vi "波形生成与数据存储.vi"(6 "文件保存控制位":bool, 9 "数据输入":i32[][](array[numeric]), 10 "上一时刻时间输入":timestamp, 11 "文件存储地址":path) -> (1 "缓存区输出":i32[][](array[numeric]), 2 "时间输出":timestamp, 3 "波形图表 6":waveform(i32)[](graph))   [LabVIEW 2020]
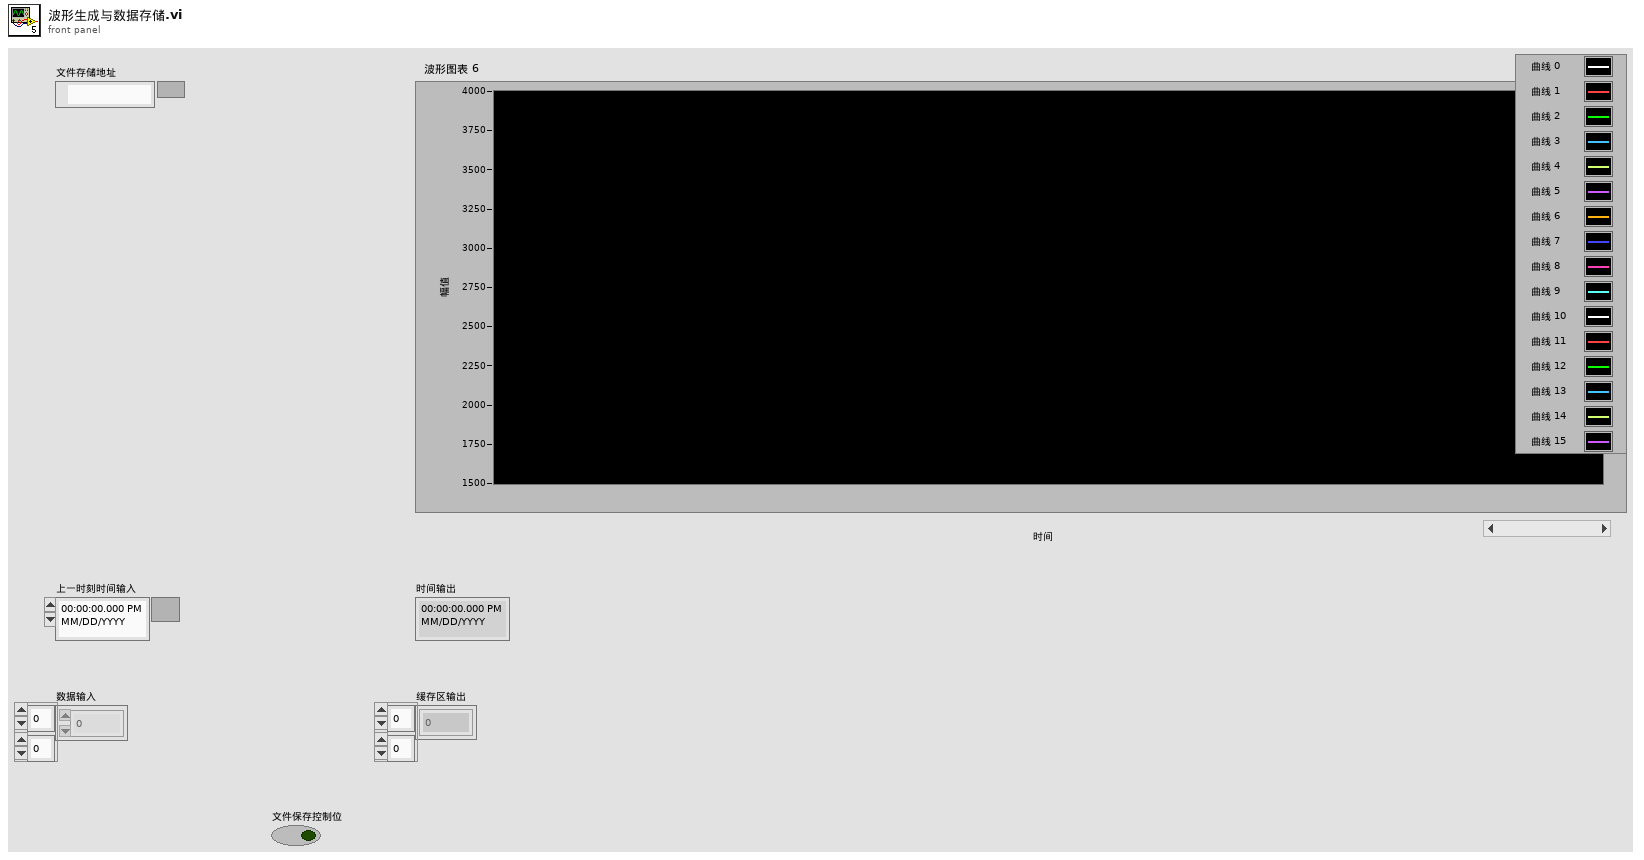
[diagram p1: front panel]
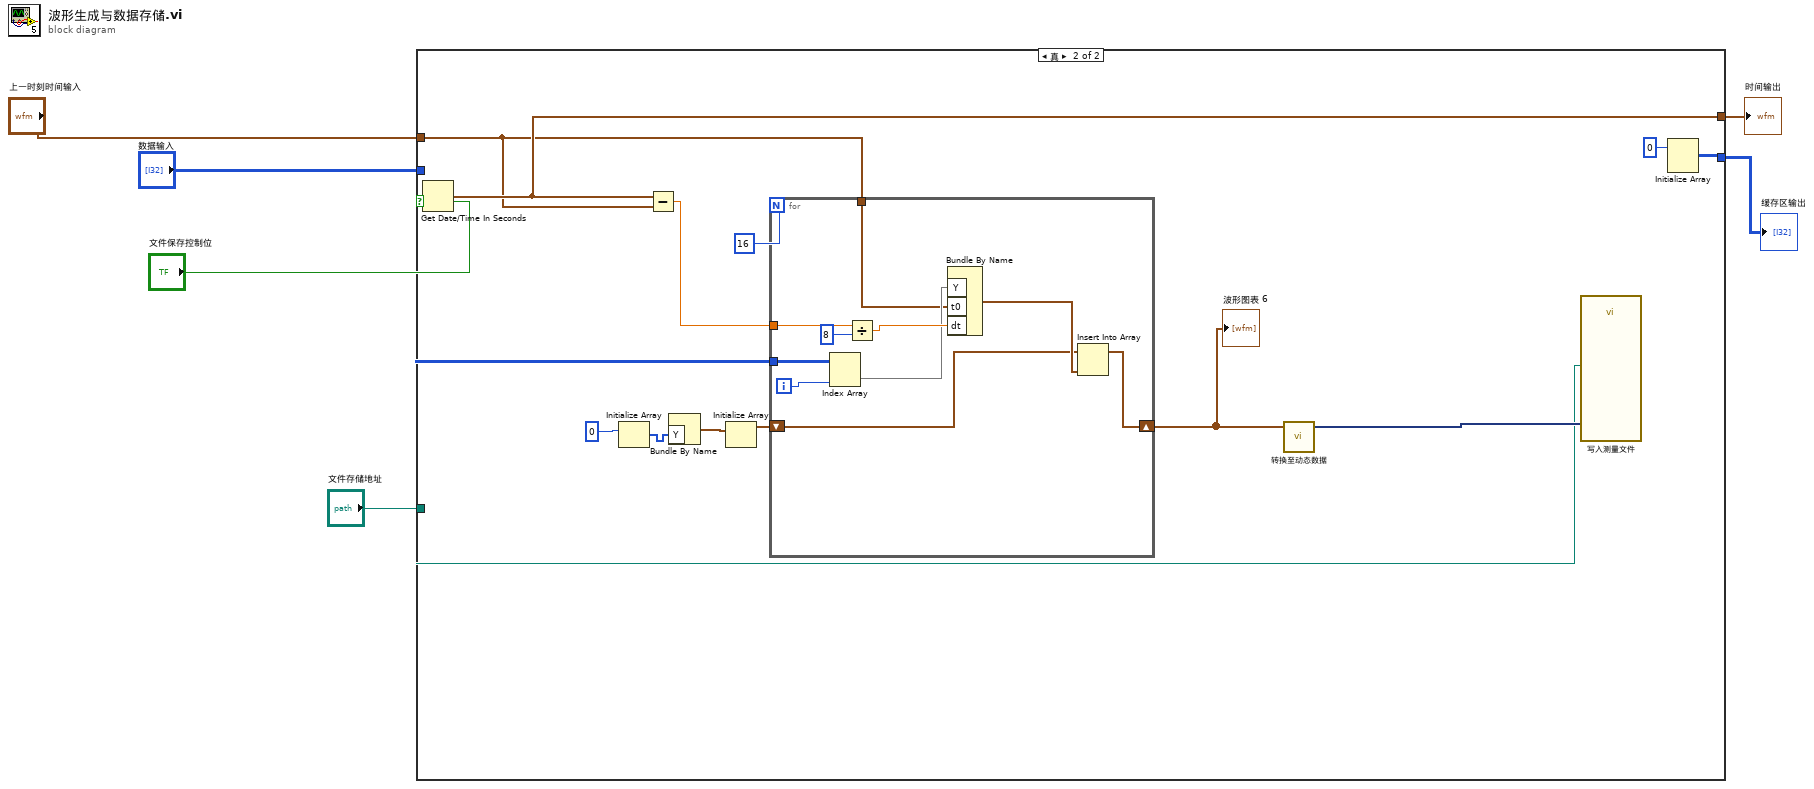
[diagram p0: block diagram]
diagram:
  n1 = case shown="真" "文件保存控制位" {
    tunnel: "数据输入" -> [w8 w12]
    tunnel: [w8 w21] -> w3
    tunnel: [w7 w11] -> w4
    tunnel: "上一时刻时间输入" -> [w7 w10]
    tunnel: "文件存储地址" -> [_ w9]
    frame False {
    }
    frame True {
      n2 = Get Date/Time In Seconds() -> (seconds since 1Jan1904=w11:timestamp)
      n3 = Initialize Array(0) -> (w16:i32[])  [unwired: 1 in]
      n4 = Subtract(x=w11, y=w10) -> (x-y=w15:dbl)
      n5 = Bundle By Name ("创建波形")("Y"=w16) -> (w18:waveform(i32))  [unwired: 1 in]
      n6 = Initialize Array(w18) -> (w19:waveform(i32)[])  [unwired: 1 in]
      n7 = for {
        N: 16 -> [_]
        shift-right: [w30] -> w14
        shift-left: w19 -> [w29]
        tunnel: w15 -> [w28]
        tunnel: w12 -> [w25]
        tunnel: w10 -> [w23]
        i -> [w32]
        n8 = Index Array(array=w25, index (col)=w32) -> (element=w24:i32[])  [unwired: 1 in]
        n9 = Divide(x=w28, y=8) -> (x/y=w27:dbl)
        n10 = Bundle By Name ("创建波形")("Y"=w24, "t0"=w23, "dt"=w27) -> (w31:waveform(i32))  [unwired: 1 in]
        n11 = Insert Into Array(array=w29, new element=w31) -> (w30:waveform(i32)[])  [unwired: 1 in]
      }
      "波形图表 6" <- w14
      n12 = call "转换至动态数据"("Array of Waveforms"=w14) -> ("Dynamic Data Type"=w13:dynamicdata)  [unwired: 3 in]
      n13 = call "写入测量文件"("Signals"=w13, "Filename"=w9) -> ()  [unwired: 15 in, 3 out]
      n14 = Initialize Array(0) -> (w21:i32[][])  [unwired: 2 in]
    }
  }
  "时间输出" <- w4
  "缓存区输出" <- w3
